vi "External Builder.vi"(11 "Arguments":string[](array[string])) -> (2 "Log String":string, 3 "Return Code":i32)   [LabVIEW 2019]
uses:
  <vilib>/AppBuilder/AB_API/common/AB_API Version Information.ctl
  <vilib>/AppBuilder/AB_API/EXE/NI_AB_API_EXE.lvclass
panel:
  out "error out":errorcluster
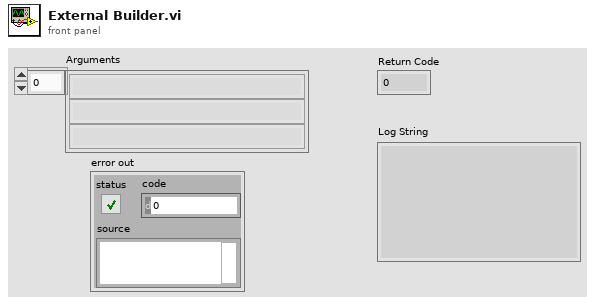
[diagram p1: front panel]
types:
  T1 = typedef "AB_API Version Information.ctl" = cluster{"Product name":string, "Legal copyright":string, "Company name":string, "Internal name":string, "File description":string}
  T2 = typedef "CLI Inputs.ctl" = cluster{"DestDir":path, "Version number":T3}
  T3 = typedef "AB_API Version Number.ctl" = cluster{"Major":u16, "Minor":u16, "Fix":u16, "Build":u16}
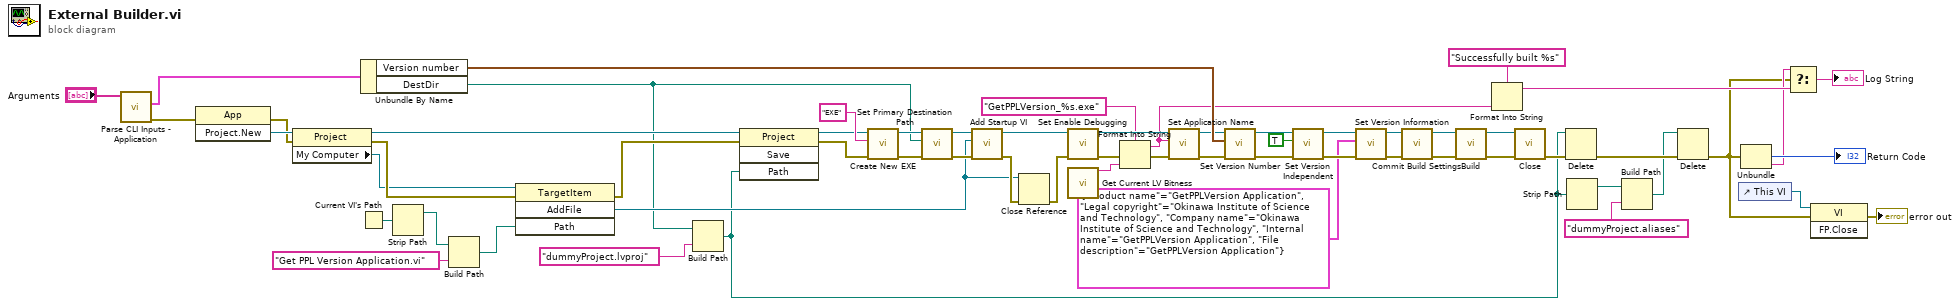
[diagram p0: block diagram]
diagram:
  n1 = call "Parse CLI Inputs - Application.vi"("Arguments"="Arguments") -> ("error out"=w50:errorcluster, "CLI Inputs"=w49:T2)  [unwired: 9 in]
  n2 = invoke class="App" method="Project.New"(error in=w50) -> (error out=w48:errorcluster, "Project:New"=w60:refnum<vi>)  [unwired: 2 in, 1 out]
  n3 = property class="Project"(reference=w60, error in=w48) -> (reference out=w21:refnum<vi>, error out=w47:errorcluster, "My Computer"=w10:refnum<vi>)
  n4 = Current VI's Path() -> (path=w46:path)
  n5 = Unbundle By Name(w49) -> ("Version number"=w61:T3, "DestDir"=w3:path)
  n6 = Strip Path(path=w46) -> (stripped path=w43:path)  [unwired: 1 out]
  n7 = Build Path(base path=w43, name or relative path="Get PPL Version Application.vi") -> (appended path=w41:path)
  n8 = invoke class="TargetItem" method="AddFile"(reference=w10, error in=w47, "Path"=w41) -> (error out=w17:errorcluster, "AddFile"=w18:refnum<vi>)  [unwired: 1 in, 2 out]
  n9 = Build Path(base path=w3, name or relative path="dummyProject.lvproj") -> (appended path=w7:path)
  n10 = invoke class="Project" method="Save"(reference=w21, error in=w17, "Path"=w7) -> (reference out=w13:refnum<vi>, error out=w12:errorcluster)  [unwired: 1 in, 2 out]
  n11 = call <vilib>:"Create New EXE.vi"("error in (no error)"=w12, "Build specification name"="EXE", "Project Refnum"=w13) -> ("error out"=w14:errorcluster, "EXE out"=w15:refnum<class "NI_AB_API_EXE.lvclass">)  [unwired: 7 in]
  n12 = call-dynamic "Set Primary Destination Path.vi"("error in (no error)"=w14, "Destination path"=w3, "Build in"=w15) -> ("error out"=w39:errorcluster, "Build out"=w40:refnum<class "NI_AB_API_EXE.lvclass">)  [unwired: 7 in]
  n13 = call-dynamic "Add Startup VI.vi"("error in (no error)"=w39, "ProjectItem Refnum"=w18, "EXE in"=w40) -> ("error out"=w37:errorcluster, "EXE out"=w38:refnum<class "NI_AB_API_EXE.lvclass">)  [unwired: 7 in]
  n14 = Close Reference(reference=w18, error in (no error)=w37) -> (error out=w19:errorcluster)
  n15 = call-dynamic "Set Enable Debugging.vi"("error in (no error)"=w19, "EXE in"=w38) -> ("error out"=w58:errorcluster, "EXE out"=w59:refnum<class "NI_AB_API_EXE.lvclass">)  [unwired: 8 in]
  n16 = call <vilib>:"Get Current LV Bitness.vi"() -> ("bitness"=w44:string)  [unwired: 11 in]
  n17 = Format Into String(format string="GetPPLVersion_%s.exe" ("Application file name"), error in=w58, w44) -> (resulting string=w1:string, error out=w45:errorcluster)  [unwired: 1 in]
  n18 = call-dynamic "Set Application Name.vi"("error in (no error)"=w45, "Application file name"=w1, "EXE in"=w59) -> ("error out"=w31:errorcluster, "EXE out"=w32:refnum<class "NI_AB_API_EXE.lvclass">)  [unwired: 7 in]
  n19 = call-dynamic "Set Version Number.vi"("error in (no error)"=w31, "Version number"=w61, "EXE in"=w32) -> ("error out"=w56:errorcluster, "EXE out"=w57:refnum<class "NI_AB_API_EXE.lvclass">)  [unwired: 7 in]
  n20 = call-dynamic "Set Version Independent.vi"("error in (no error)"=w56, "versionIndependent"=TRUE, "NI_AB_API_EXE in"=w57) -> ("error out"=w54:errorcluster, "NI_AB_API_EXE out"=w55:refnum<class "NI_AB_API_EXE.lvclass">)  [unwired: 7 in]
  n21 = call-dynamic "Set Version Information.vi"("error in (no error)"=w54, "Version Information"=T1 {"Product name"="GetPPLVersion Application", "Legal copyright"="Okinawa Institute of Science and Technology", "Company name"="Okinawa Institute of Science and Technology", "Internal name"="GetPPLVersion Application", "File description"="GetPPLVersion Application"}, "NI_AB_API_EXE in"=w55) -> ("error out"=w35:errorcluster, "NI_AB_API_EXE out"=w36:refnum<class "NI_AB_API_EXE.lvclass">)  [unwired: 7 in]
  n22 = call-dynamic "Commit Build Settings.vi"("error in (no error)"=w35, "EXE in"=w36) -> ("error out"=w33:errorcluster, "EXE out"=w34:refnum<class "NI_AB_API_EXE.lvclass">)  [unwired: 8 in]
  n23 = call-dynamic "Build.vi"("error in (no error)"=w33, "EXE in"=w34) -> ("error out"=w52:errorcluster, "EXE out"=w53:refnum<class "NI_AB_API_EXE.lvclass">)  [unwired: 6 in, 2 out]
  n24 = Format Into String(format string="Successfully built %s", w1) -> (resulting string=w24:string)  [unwired: 2 in, 1 out]
  n25 = call-dynamic "Close.vi"("error in (no error)"=w52, "EXE in"=w53) -> ("error out"=w25:errorcluster)  [unwired: 9 in]
  n26 = Delete(path (use dialog)=w7, error in=w25) -> (error out=w8:errorcluster)  [unwired: 3 in, 2 out]
  n27 = Strip Path(path=w7) -> (stripped path=w6:path)  [unwired: 1 out]
  n28 = Build Path(base path=w6, name or relative path="dummyProject.aliases") -> (appended path=w5:path)
  n29 = Delete(path (use dialog)=w5, error in=w8) -> (error out=w9:errorcluster)  [unwired: 3 in, 2 out]
  n30 = control-ref of="This VI"() -> (w28:refnum<vi>)
  n31 = Unbundle(w9) -> ("code"=→"Return Code":i32, "source"=w23:string)  [unwired: 1 out]
  n32 = Select(t=w23, s=w9, f=w24) -> (s? t:f=→"Log String":string)
  n33 = invoke class="VI" method="FP.Close"(reference=w28, error in=w9) -> (error out=→"error out":errorcluster)  [unwired: 1 in, 2 out]
